vi "PII_Controller_1SDI_v00.vi"(8 "Integrator (-1)":i32, 9 "PII out (-1)":i16, 10 "Control Cavity":T1={"Lock"=FALSE, "Hold"=FALSE, "P Gain"=0, "P BS"=-5, "I Gain"=0, "I BS"=-10, "I2 G"=0, "I2 BS"=-26, "Scan Amp"=0, "Scan Off"=0, "Scan FS"=0, "SFS BS"=0, "I Max value"=10000, "I2 Max value"=10000, "Scope.Offset"=0, "Trigger Direction"=enum."either", "Scan-PII thresh"=0}, 11 "OPO A Error":i16) -> (0 "I Cavity":i32, 1 "PII out":i16, 3 "I too high?":bool)   [LabVIEW 2013]
doc: "This is a PII Controller used here to lock cavities. Pound-Drever-Hall error signals are fed in and the PII output is fed out. Designed by Seiji Armstrong, based on a design by Ben Sparkes."
uses:
  Strict Type Defs/PII individual.ctl
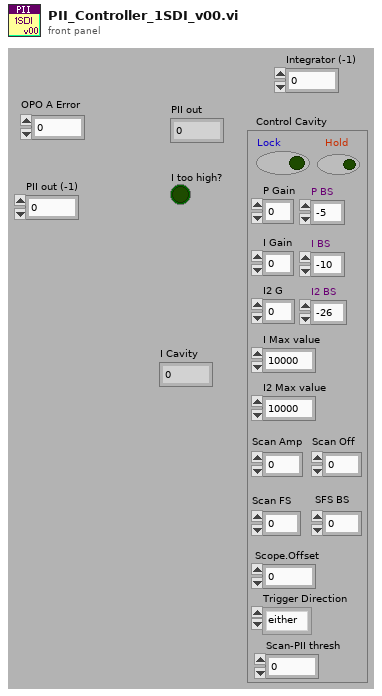
[diagram p1: front panel]
types:
  T1 = typedef "PII individual.ctl" = cluster{"Lock":bool, "Hold":bool, "P Gain":i32, "P BS":i16, "I Gain":i32, "I BS":i16, "I2 G":i32, "I2 BS":i16, "Scan Amp":i16, "Scan Off":i16, "Scan FS":u16, "SFS BS":i16, "I Max value":i32, "I2 Max value":i32, "Scope.Offset":i16, "Trigger Direction":enum8{"either", "minus-plus", "plus-minus"}, "Scan-PII thresh":i16}
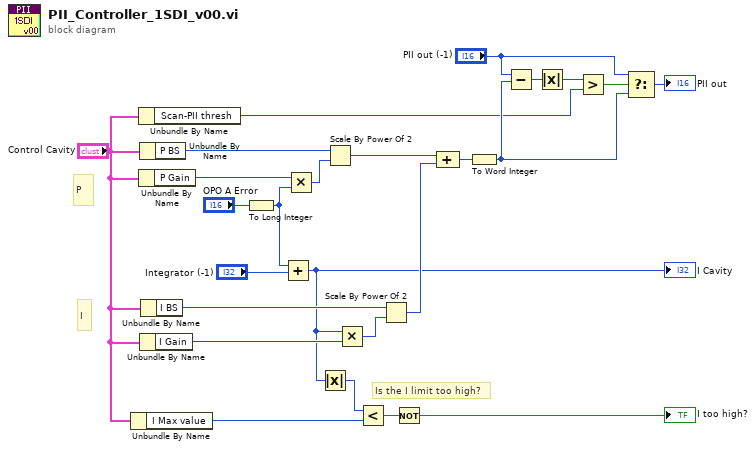
[diagram p0: block diagram]
diagram:
  # "Is the I limit too high?"
  # "P"
  # "I"
  n1 = Unbundle By Name("Control Cavity") -> ("I Max value"=w15:i32)
  n2 = Unbundle By Name("Control Cavity") -> ("Scan-PII thresh"=w4:i16)
  n3 = Unbundle By Name("Control Cavity") -> ("P Gain"=w17:i32)
  n4 = Unbundle By Name("Control Cavity") -> ("P BS"=w23:i16)
  n5 = Unbundle By Name("Control Cavity") -> ("I Gain"=w22:i32)
  n6 = Unbundle By Name("Control Cavity") -> ("I BS"=w21:i16)
  n7 = To Long Integer(number="OPO A Error") -> (32bit integer=w12:i32)
  n8 = Add(x=w12, y="Integrator (-1)") -> (x+y=w2:i32)
  "I Cavity" <- w2
  n9 = Multiply(x=w17, y=w12) -> (x*y=w24:i32)
  n10 = Absolute Value(x=w2) -> (abs(x)=w25:i32)
  n11 = Scale By Power Of 2(n=w23, x=w24) -> (x*2^n=w18:i32)
  n12 = Multiply(x=w2, y=w22) -> (x*y=w20:i32)
  n13 = Less?(x=w25, y=w15) -> (x < y?=w3:bool)
  n14 = Scale By Power Of 2(n=w21, x=w20) -> (x*2^n=w19:i32)
  n15 = Not(x=w3) -> (.not. x?=→"I too high?":bool)
  n16 = Compound Arithmetic op=ADD(w18, w19) -> (w11:i32)
  n17 = To Word Integer(number=w11) -> (16bit integer=w8:i16)
  n18 = Subtract(x="PII out (-1)", y=w8) -> (x-y=w10:i16)
  n19 = Absolute Value(x=w10) -> (abs(x)=w5:i16)
  n20 = Greater?(x=w5, y=w4) -> (0:w9:bool)
  n21 = Select(t="PII out (-1)", s=w9, f=w8) -> (s? t:f=→"PII out":i16)
